vi "Get Item by name array.vi"(8 "error in (no error)":errorcluster, 10 "Name Array":string[](array[string]), 11 "JSON Value In":refnum<class "JSON Value.lvclass">) -> (0 "error out":errorcluster, 1 "found":bool, 2 "Value":refnum<class "JSON Value.lvclass">, 3 "JSON Value Out":refnum<class "JSON Value.lvclass">)   [LabVIEW 2020, in "Library Commun.lvlib" / "JSON Value.lvclass"]
doc: "Gets a JSON Value from a JSON collection by it's path. The paths is an array of strings.\nThe first element is the top level name. For elements in an array you can use a %d formatted number to index an element out.\n\nCopyright 2012 James David Powell, Shaun Rumbell and Ton Plomp\nMore information on http://lavag.org/topic/16217-cr-json-labview"
uses:
  JSON Value.lvclass
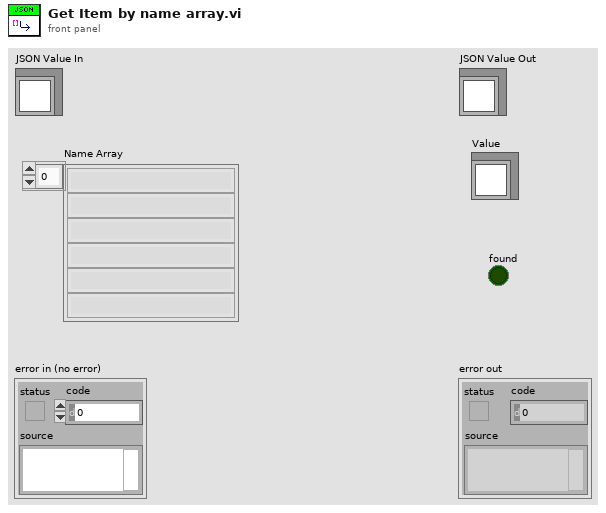
[diagram p1: front panel]
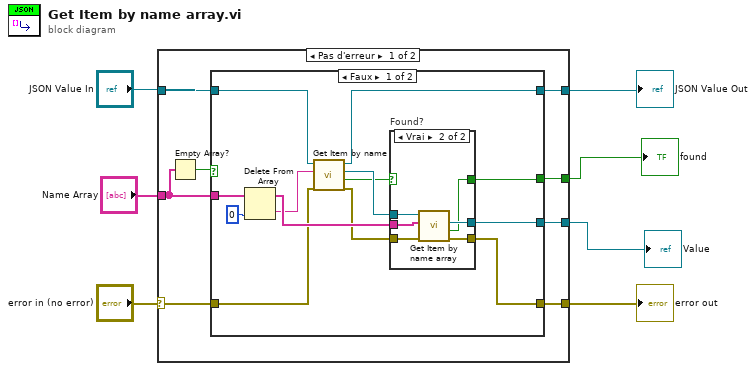
[diagram p0: block diagram]
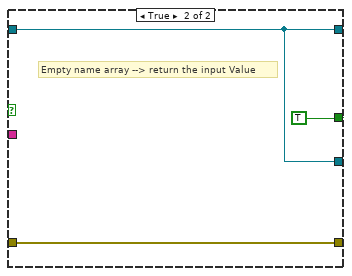
[diagram p3: hidden frame]
diagram:
  n1 = case shown="Pas d'erreur" "error in (no error)" {
    selector: "error in (no error)" -> [w13 w42]
    tunnel: [w12 w42] -> w4
    tunnel: [w14 w41] -> w6
    tunnel: "JSON Value In" -> [w15 w41]
    tunnel: "Name Array" -> [w9 _]
    tunnel: [w11 _] -> w2
    tunnel: [w10 _] -> w1
    frame No Error {
      n2 = Empty Array?(array=w9) -> (empty?=w8:bool)
      n3 = case shown="Faux" w8 {
        tunnel: w15 -> [w23 w40]
        tunnel: [w22 w40] -> w14
        tunnel: w13 -> [w21 w38]
        tunnel: [w20 w38] -> w12
        tunnel: [w19 w40] -> w11
        tunnel: [w18 TRUE ("found")] -> w10
        tunnel: w9 -> [w17 _]
        frame False {
          n4 = Delete From Array(array=w17, index=0) -> (deleted portion=w24:string, array with subset deleted=w26:string[])  [unwired: 1 in]
          n5 = call-dynamic "Get Item by name.vi"("error in (no error)"=w21, "name"=w24, "JSON Value In"=w23) -> ("error out"=w25:errorcluster, "found"=w16:bool, "Value"=w27:refnum<class "JSON Value.lvclass">, "JSON Value Out"=w22:refnum<class "JSON Value.lvclass">)  [unwired: 5 in]
          n6 = case "Found?" shown="Vrai" w16 {
            selector: w16 -> [w29 _]
            tunnel: w27 -> [w30 w37]
            tunnel: w26 -> [_ w36]
            tunnel: [w29 w32] -> w18
            tunnel: [w30 w33] -> w19
            tunnel: w25 -> [w31 w35]
            tunnel: [w31 w34] -> w20
            frame False {
            }
            frame True {
              n7 = call "Get Item by name array.vi"("error in (no error)"=w35, "Name Array"=w36, "JSON Value In"=w37) -> ("error out"=w34:errorcluster, "found"=w32:bool, "Value"=w33:refnum<class "JSON Value.lvclass">)  [unwired: 5 in, 1 out]
            }
          }
        }
        frame True {
          # "Empty name array --> return the input Value"
        }
      }
    }
    frame Error {
    }
  }
  "error out" <- w4
  "JSON Value Out" <- w6
  "found" <- w1
  "Value" <- w2
